vi "MAIN.vi"() -> ()   [LabVIEW 2011]
uses:
  <vilib>/Utility/file.llb/Read From Spreadsheet File (string).vi
panel:
  out "State buffer":string
  in  "Reset":bool
  in  "State":bool
  in  "Data":bool
  in  "file path (use dialog)":path=path "C:/tyrmt/data.csv.txt"
  in  "VISA resource name":refnum<visa-resource-name>="COM4"
  in  "Tab Control":T1(tab)
  out "FFT Phi/Roll Gyro X":dbl[](graph)
  out "FFT Theta/Pitch Gyro Y":dbl[](graph)
  out "FFT Psi/Yaw Gyro Z":dbl[](graph)
  out "FFT Az":dbl[](graph)
  out "FFT Ay":dbl[](graph)
  out "FFT Ax":dbl[](graph)
  out "Velocity X direction":dbl[](graph)
  out "Velocity Y direction":dbl[](graph)
  out "Velocity Z direction":dbl[](graph)
  out "min velocity Y direction":dbl
  out "max velocity Y direction":dbl
  out "min velocity X direction":dbl
  out "max velocity X direction":dbl
  out "min velocity Z direction":dbl
  out "max velocity Z direction":dbl
  out "Az":dbl[](array[numeric])
  out "Ay":dbl[](array[numeric])
  out "Ax":dbl[](array[numeric])
  out "gz":dbl[](array[numeric])
  out "gy":dbl[](array[numeric])
  out "gx":dbl[](array[numeric])
  out "Z Accelerometer":dbl[](array[numeric])
  out "Y Accelerometer":dbl[](array[numeric])
  out "X Accellerometer":dbl[](array[numeric])
  out "Psi/Yaw Gyro Z":dbl[](array[numeric])
  out "Theta/Pitch Gyro Y":dbl[](array[numeric])
  out "Phi/Roll Gyro X":dbl[](array[numeric])
  out "Psi from quaternions":dbl[](array[numeric])
  out "Theta from quaternions":dbl[](array[numeric])
  out "Phi from quaternions":dbl[](array[numeric])
  in  "Load in CSV File":path
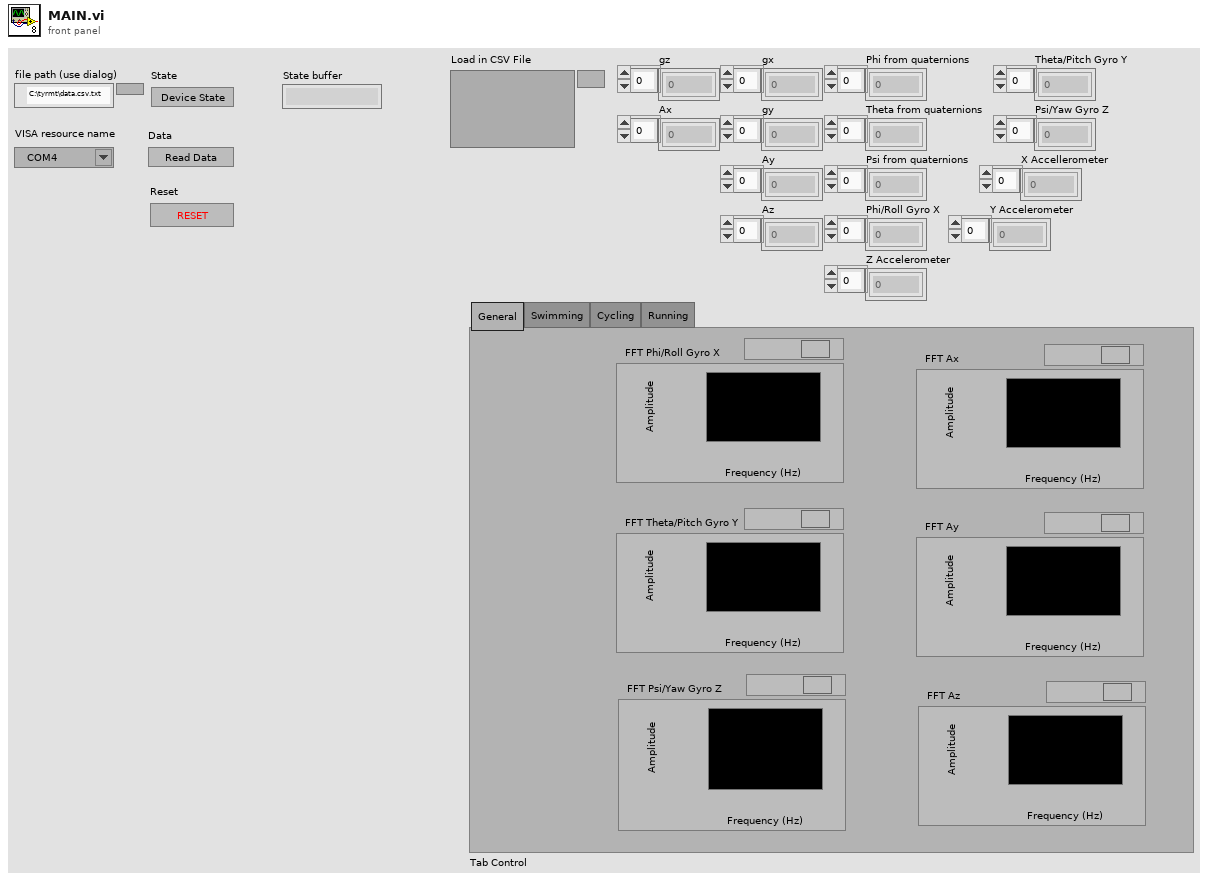
[diagram p1: front panel]
types:
  T1 = enum32{"General", "Swimming", "Cycling", "Running"}
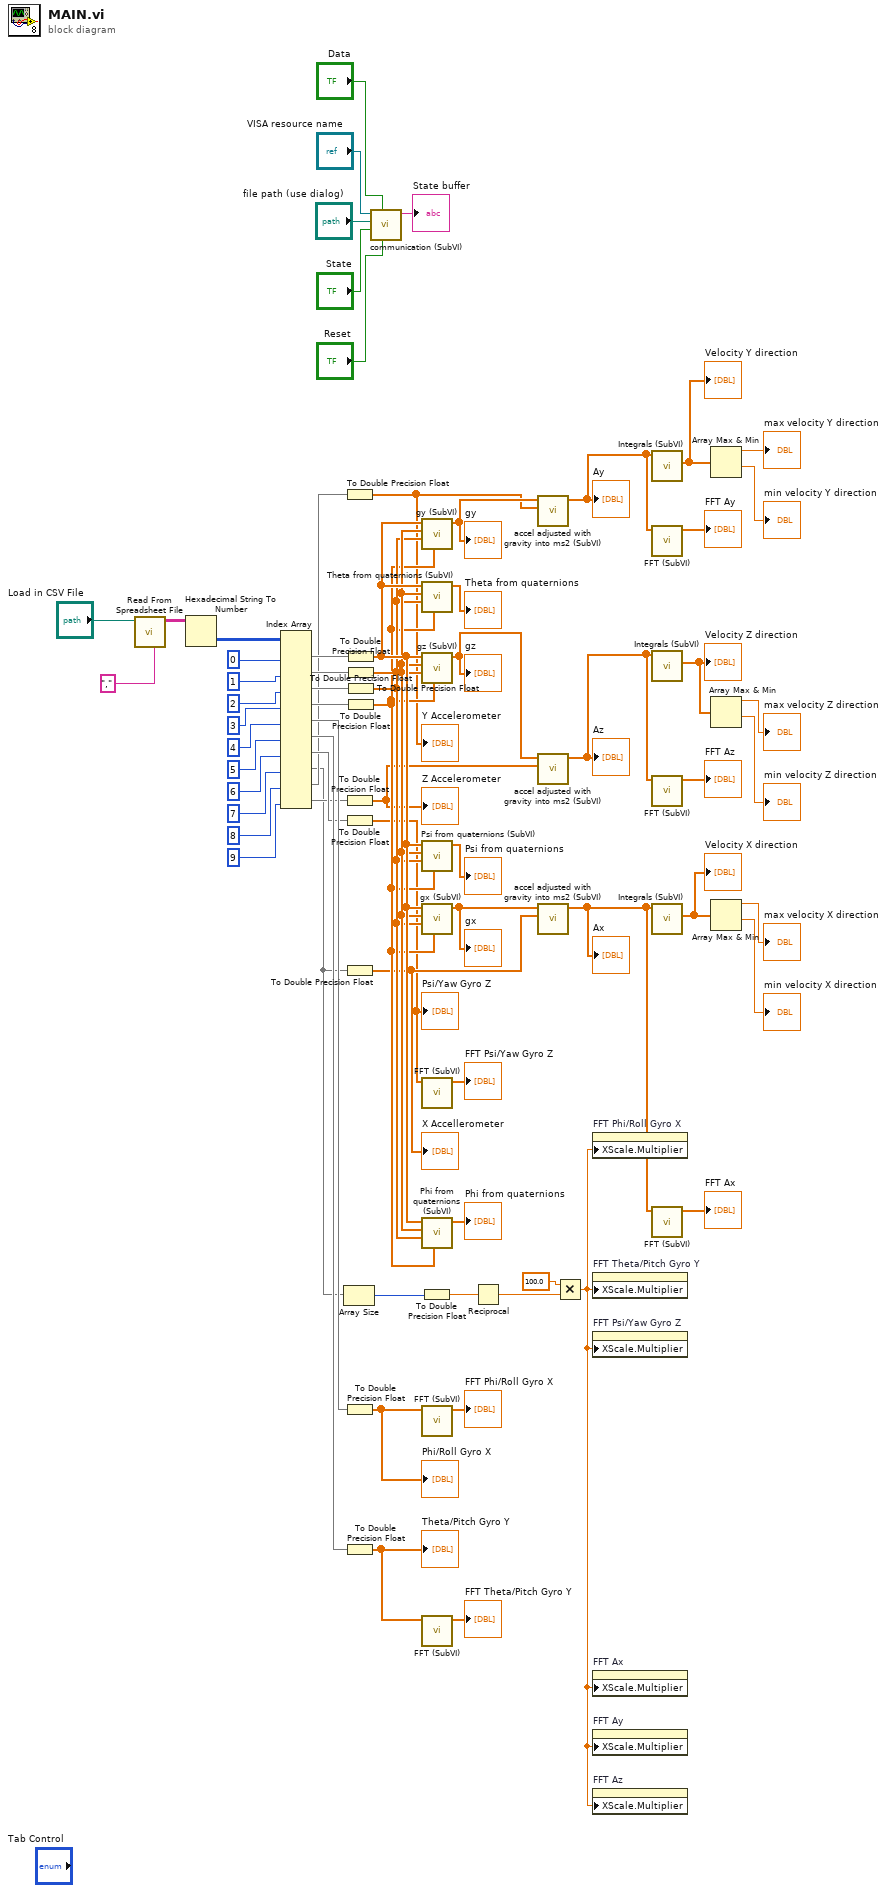
[diagram p0: block diagram]
diagram:
  n1 = call-poly <vilib>:"Read From Spreadsheet File.vi"("delimiter (\\t)"="," ("delimiter (\\t)"), "file path (dialog if empty)"="Load in CSV File") -> ("all rows"=w67:string[][])  [unwired: 5 in, 4 out]
  n2 = Hexadecimal String To Number(string=w67) -> (number=w66:u32[][])  [unwired: 2 in, 1 out]
  n3 = Index Array(array=w66, index (col) #1=0 ("disabled index (col)"), index (col) #2=1 ("index (col)"), index (col) #3=2 ("index (col)"), index (col) #4=3 ("index (col)"), index (col) #5=4 ("index (col)"), index (col) #6=5 ("index (col)"), index (col) #7=6 ("index (col)"), index (col) #8=7 ("index (col)"), index (col) #9=8 ("index (col)"), index (col) #10=9 ("index (col)")) -> (element #1=w55:u32[], element #2=w54:u32[], element #3=w53:u32[], element #4=w52:u32[], element #5=w48:u32[], element #6=w47:u32[], element #7=w46:u32[], element #8=w23:u32[], element #9=w45:u32[], element #10=w44:u32[])  [unwired: 10 in]
  n4 = Array Size(array=w23) -> (size(s)=w19:i32)
  n5 = To Double Precision Float(number=w45) -> (double precision float=w35:dbl[])
  "Y Accelerometer" <- w35
  n6 = To Double Precision Float(number=w44) -> (double precision float=w34:dbl[])
  "Z Accelerometer" <- w34
  n7 = To Double Precision Float(number=w46) -> (double precision float=w32:dbl[])
  "Psi/Yaw Gyro Z" <- w32
  n8 = To Double Precision Float(number=w23) -> (double precision float=w33:dbl[])
  "X Accellerometer" <- w33
  n9 = To Double Precision Float(number=w48) -> (double precision float=w43:dbl[])
  "Phi/Roll Gyro X" <- w43
  n10 = To Double Precision Float(number=w47) -> (double precision float=w31:dbl[])
  "Theta/Pitch Gyro Y" <- w31
  n11 = To Double Precision Float(number=w55) -> (double precision float=w42:dbl[])
  n12 = To Double Precision Float(number=w54) -> (double precision float=w41:dbl[])
  n13 = To Double Precision Float(number=w53) -> (double precision float=w40:dbl[])
  n14 = To Double Precision Float(number=w52) -> (double precision float=w39:dbl[])
  n15 = call "communication (SubVI).vi"("Reset"="Reset", "Data"="Data", "State"="State", "file path (use dialog)"="file path (use dialog)", "VISA Refnum in"="VISA resource name") -> ("State buffer"=→"State buffer":string)  [unwired: 6 in]
  n16 = call "gy (SubVI).vi"("Array in"=w39, "Array 3"=w40, "Array 4"=w41, "Array 5"=w42) -> ("Array out"=w37:dbl[])  [unwired: 7 in]
  "gy" <- w37
  n17 = call "Theta from quaternions (SubVI).vi"("Array 3"=w39, "Array 4"=w40, "Array in"=w41, "Array 5"=w42) -> ("Array out"=→"Theta from quaternions":dbl[])  [unwired: 7 in]
  n18 = call "gz (SubVI).vi"("Array in"=w39, "Array 3"=w40, "Array 4"=w41, "Array 5"=w42) -> ("Array out"=w36:dbl[])  [unwired: 7 in]
  "gz" <- w36
  n19 = call "Psi from quaternions (SubVI).vi"("Array in"=w39, "Array 3"=w40, "Array 4"=w41, "Array 5"=w42) -> ("Array out"=→"Psi from quaternions":dbl[])  [unwired: 7 in]
  n20 = call "gx (SubVI).vi"("Array 4"=w39, "Array in"=w40, "Array 5"=w41, "Array 3"=w42) -> ("Array out"=w38:dbl[])  [unwired: 7 in]
  "gx" <- w38
  n21 = call "FFT (SubVI).vi"("Array in"=w32) -> ("Array out"=→"FFT Psi/Yaw Gyro Z":dbl[])  [unwired: 10 in]
  n22 = call "Phi from quaternions (SubVI).vi"("Array in"=w39, "Array 3"=w40, "Array 4"=w41, "Array 5"=w42) -> ("Array out"=→"Phi from quaternions":dbl[])  [unwired: 7 in]
  n23 = To Double Precision Float(number=w19) -> (double precision float=w20:dbl)
  n24 = call "FFT (SubVI).vi"("Array in"=w43) -> ("Array out"=→"FFT Phi/Roll Gyro X":dbl[])  [unwired: 10 in]
  n25 = call "FFT (SubVI).vi"("Array in"=w31) -> ("Array out"=→"FFT Theta/Pitch Gyro Y":dbl[])  [unwired: 10 in]
  n26 = Reciprocal(x=w20) -> (1/x=w21:dbl)
  n27 = call "accel adjusted with gravity into ms2 (SubVI).vi"("Array in"=w35, "Array out"=w37) -> ("Array out"=w16:dbl[])  [unwired: 9 in]
  "Ay" <- w16
  n28 = call "accel adjusted with gravity into ms2 (SubVI).vi"("Array in"=w34, "Array out"=w36) -> ("Array out"=w24:dbl[])  [unwired: 9 in]
  "Az" <- w24
  n29 = call "accel adjusted with gravity into ms2 (SubVI).vi"("Array in"=w33, "Array out"=w38) -> ("Array out"=w17:dbl[])  [unwired: 9 in]
  "Ax" <- w17
  n30 = Multiply(x=100.0 ("double precision float"), y=w21) -> (x*y=w18:dbl)
  n31 = property on="FFT Phi/Roll Gyro X" class="WFGraph (strict)"("XScale.Multiplier"=w18) -> ()  [unwired: 2 in, 2 out]
  n32 = property on="FFT Theta/Pitch Gyro Y" class="WFGraph (strict)"("XScale.Multiplier"=w18) -> ()  [unwired: 2 in, 2 out]
  n33 = property on="FFT Psi/Yaw Gyro Z" class="WFGraph (strict)"("XScale.Multiplier"=w18) -> ()  [unwired: 2 in, 2 out]
  n34 = property on="FFT Ax" class="WFGraph (strict)"("XScale.Multiplier"=w18) -> ()  [unwired: 2 in, 2 out]
  n35 = property on="FFT Ay" class="WFGraph (strict)"("XScale.Multiplier"=w18) -> ()  [unwired: 2 in, 2 out]
  n36 = property on="FFT Az" class="WFGraph (strict)"("XScale.Multiplier"=w18) -> ()  [unwired: 2 in, 2 out]
  n37 = call "Integrals (SubVI).vi"("Array out"=w16) -> ("Velocity X"=w13:dbl[])  [unwired: 9 in, 1 out]
  "Velocity Y direction" <- w13
  n38 = call "FFT (SubVI).vi"("Array in"=w16) -> ("Array out"=→"FFT Ay":dbl[])  [unwired: 10 in]
  n39 = call "Integrals (SubVI).vi"("Array out"=w24) -> ("Velocity X"=w15:dbl[])  [unwired: 9 in, 1 out]
  "Velocity Z direction" <- w15
  n40 = call "FFT (SubVI).vi"("Array in"=w24) -> ("Array out"=→"FFT Az":dbl[])  [unwired: 10 in]
  n41 = call "Integrals (SubVI).vi"("Array out"=w17) -> ("Velocity X"=w14:dbl[])  [unwired: 9 in, 1 out]
  "Velocity X direction" <- w14
  n42 = call "FFT (SubVI).vi"("Array in"=w17) -> ("Array out"=→"FFT Ax":dbl[])  [unwired: 10 in]
  n43 = Array Max & Min(array=w13) -> (max value=→"max velocity Y direction":dbl, min value=→"min velocity Y direction":dbl)  [unwired: 2 out]
  n44 = Array Max & Min(array=w15) -> (max value=→"max velocity Z direction":dbl, min value=→"min velocity Z direction":dbl)  [unwired: 2 out]
  n45 = Array Max & Min(array=w14) -> (max value=→"max velocity X direction":dbl, min value=→"min velocity X direction":dbl)  [unwired: 2 out]
